vi "copy.vi"(8 "error in (no error)":errorcluster, 11 "TestCase in":refnum<class "TestCase.Pointer.lvclass">) -> (0 "error out":errorcluster, 3 "TestCase out":refnum<class "TestCase.Pointer.lvclass">)   [LabVIEW 2016, in "TestCase.Pointer.lvclass"]
uses:
  TestCase.Pointer.lvclass
  <vilib>/addons/_JKI Toolkits/VI Tester/TestCase.llb/TestCase.lvclass
  C:/Program Files (x86)/National Instruments/LabVIEW 2016/vi.lib/addons/_JKI Toolkits/VI Tester/TestCase.llb/TestCase.lvclass
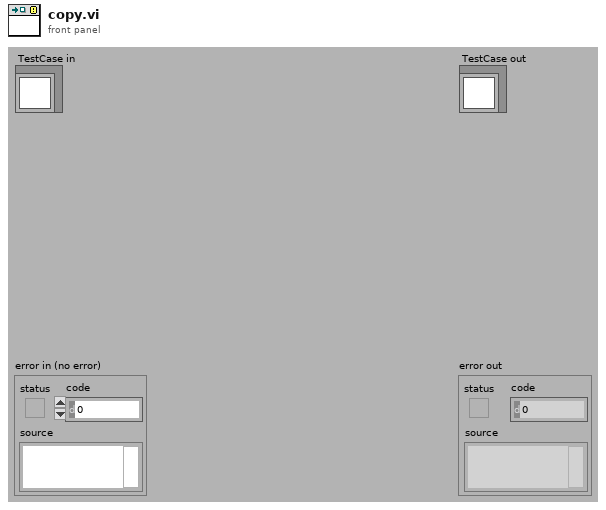
[diagram p1: front panel]
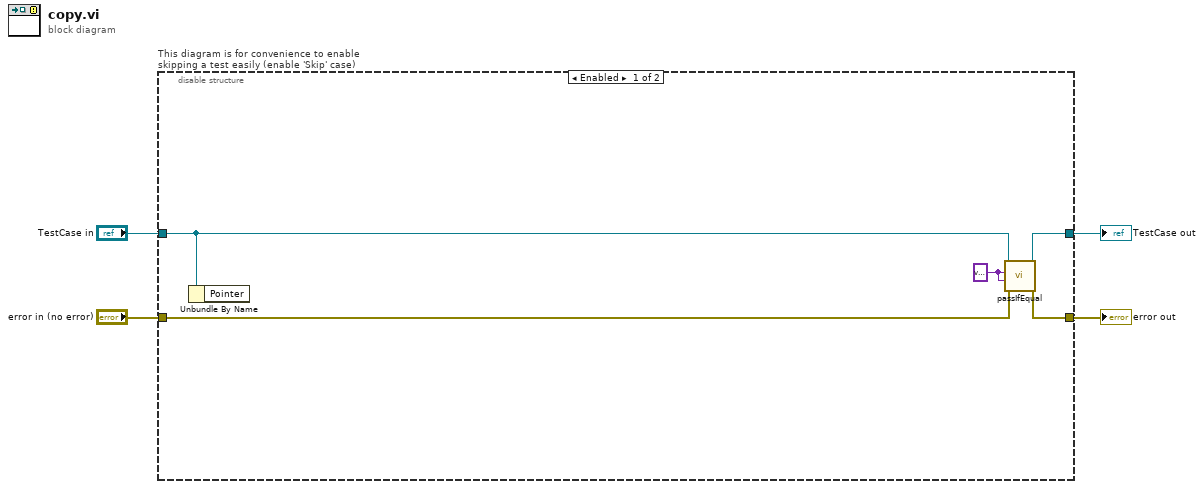
[diagram p0: block diagram]
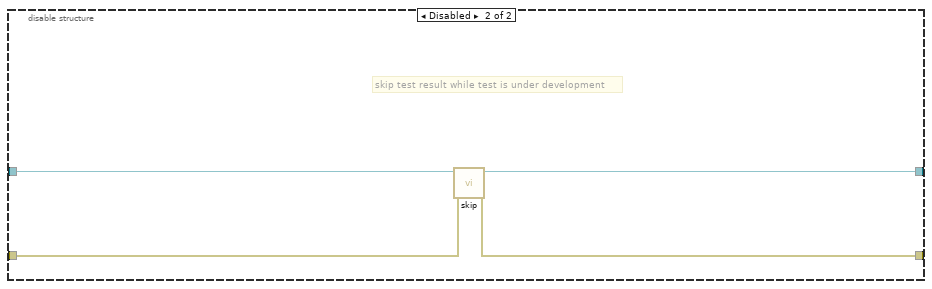
[diagram p2: hidden frame]
diagram:
  n1 = disable-structure "This diagram is for convenience to enable skipping a test easily (enable 'Skip' case)" shown="Enabled" {
    disable-tunnel: "TestCase in" -> [w7 w13]
    disable-tunnel: [w9 w11] -> w1
    disable-tunnel: [w8 w12] -> w3
    disable-tunnel: "error in (no error)" -> [w6 w10]
    frame Enabled {
      w5 = variant ("x")
      n2 = Unbundle By Name(w7) -> ()  [unwired: 1 out]
      n3 = call-dynamic "passIfEqual.vi"("error in (no error)"=w6, "y"=w5, "x"=w5, "TestCase in"=w7) -> ("error out"=w8:errorcluster, "TestCase out"=w9:refnum<class "TestCase.Pointer.lvclass">)  [unwired: 6 in]
    }
    frame Disabled {
      # "skip test result while test is under development"
      n4 = call <vilib>:"skip.vi"("error in (no error)"=w10, "TestCase in"=w13) -> ("error out"=w12:errorcluster, "TestCase out"=w11:refnum<class "TestCase.Pointer.lvclass">)  [unwired: 8 in]
    }
  }
  "error out" <- w3
  "TestCase out" <- w1
